vi "Convert QD Object String to 2D Array - Backup.vi"(11 "objects string":string) -> (2 "already sorted":bool, 3 "objects 2D array":string[][](array[string]))   [LabVIEW 2024]
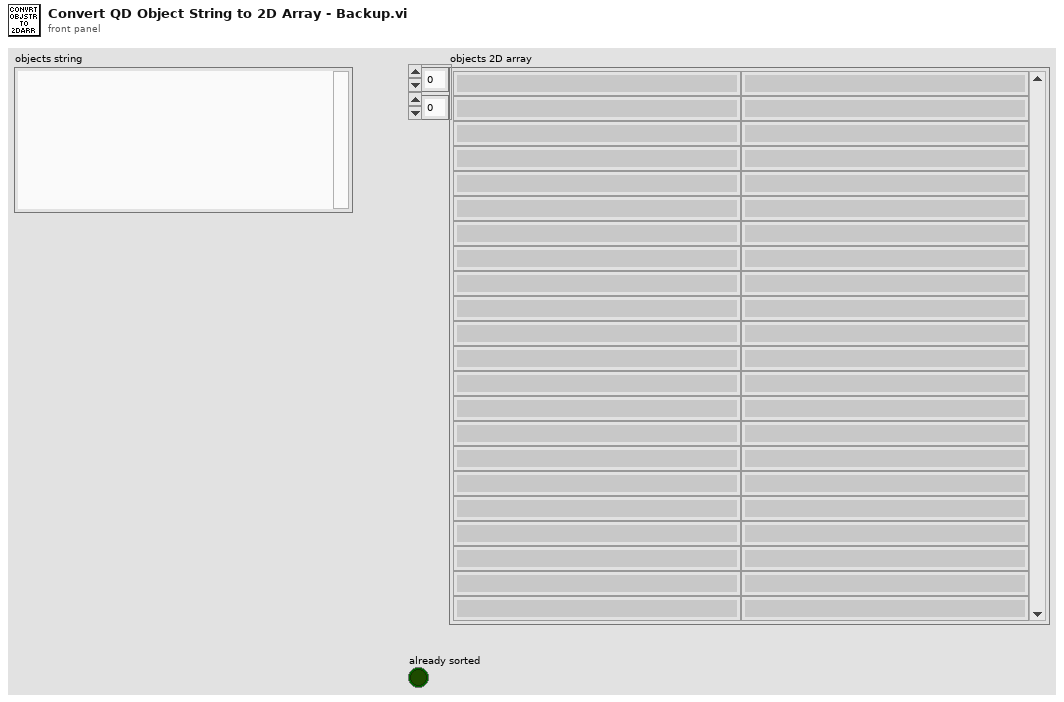
[diagram p1: front panel]
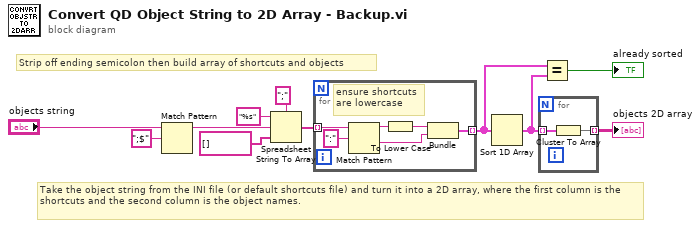
[diagram p0: block diagram]
diagram:
  # "Take the object string from the INI file (or default shortcuts file) and turn it into a 2D array, where the first column is the shortcuts and the second column is the object names."
  # "Strip off ending semicolon then build array of shortcuts and objects"
  n1 = Match Pattern(string="objects string", regular expression=";$") -> (before substring=w10:string)  [unwired: 1 in, 3 out]
  n2 = Spreadsheet String To Array(delimiter (Tab)=";", format string="%s", spreadsheet string=w10, array type (2D Dbl)=string[] []) -> (array=w6:string[])
  n3 = for {
    tunnel: w6 -> [w17] mode=indexing
    tunnel: [w12] -> w3 mode=indexing
    # "ensure shortcuts\nare lowercase"
    n4 = Match Pattern(string=w17, regular expression=":") -> (before substring=w15:string, after substring=w13:string)  [unwired: 1 in, 2 out]
    n5 = To Lower Case(string=w15) -> (all lower case string=w14:string)
    n6 = Bundle(w14, w13) -> (w12:cluster{string, string})  [unwired: 1 in]
  }
  n7 = Sort 1D Array(array=w3) -> (sorted array=w2:cluster{string, string}[])
  n8 = for {
    tunnel: w2 -> [w19] mode=indexing
    tunnel: [w18] -> w11 mode=indexing
    n9 = Cluster To Array(cluster=w19) -> (array=w18:string[])
  }
  "objects 2D array" <- w11
  n10 = Equal?(x=w3, y=w2) -> (x = y?=→"already sorted":bool)
